vi "fgv_status-display.vi"(7 "Mode":T1=enum."Update", 8 "error in":errorcluster, 9 "detail":string, 10 "title":string, 11 "System Log":refnum<vi>) -> (0 "error out":errorcluster)   [LabVIEW 2019]
uses:
  _ctrl/system-status.ctl
panel:
  out "deleted portion":string[](array[string])
  out "concatenated string":string
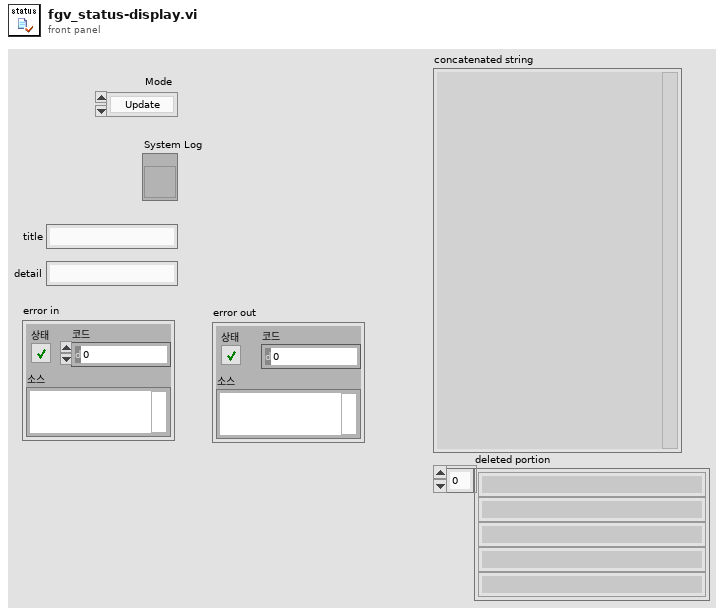
[diagram p1: front panel]
types:
  T1 = typedef "system-status.ctl" = enum16{"Initial", "Update", "Clear", "Read"}
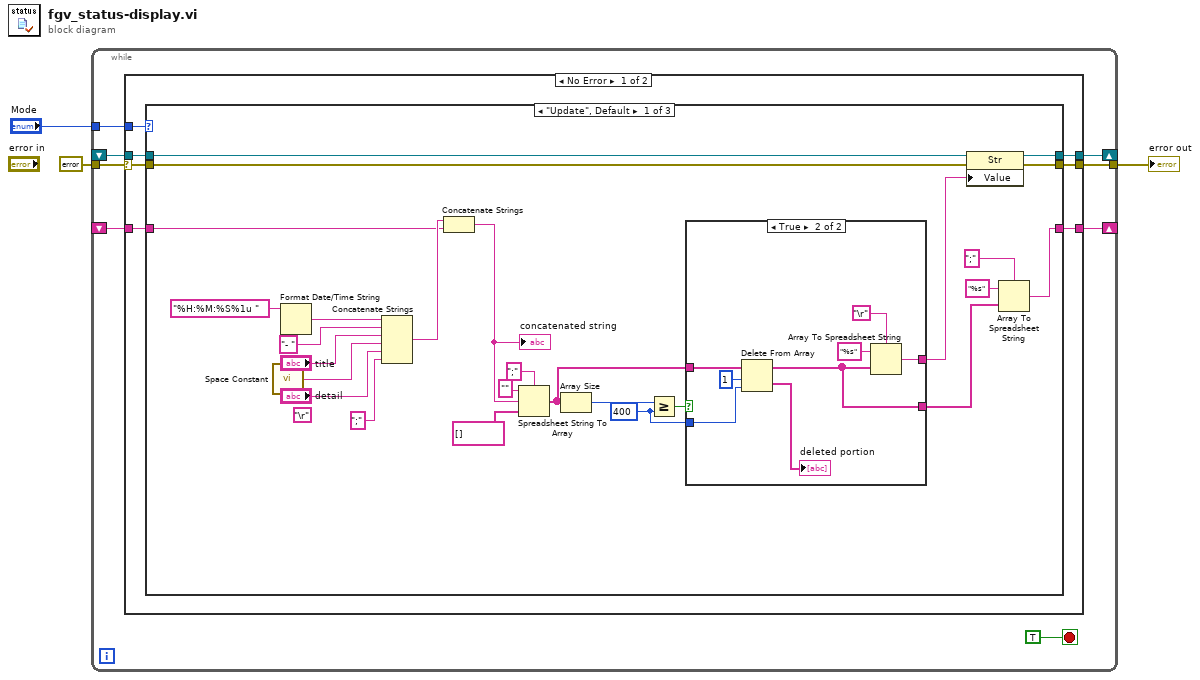
[diagram p0: block diagram]
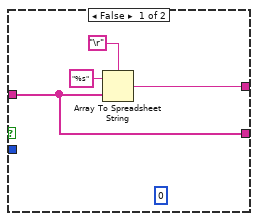
[diagram p2: hidden frame]
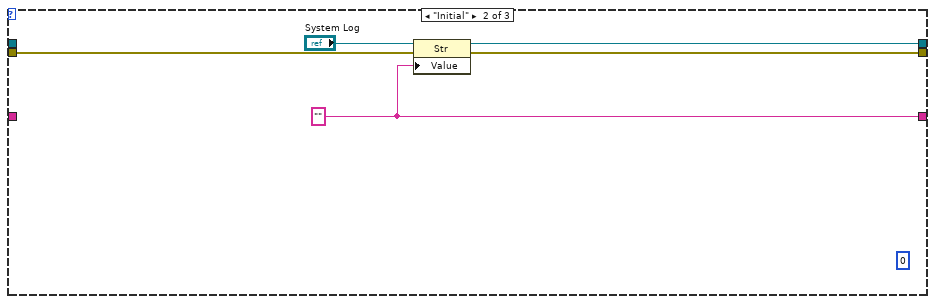
[diagram p3: hidden frame]
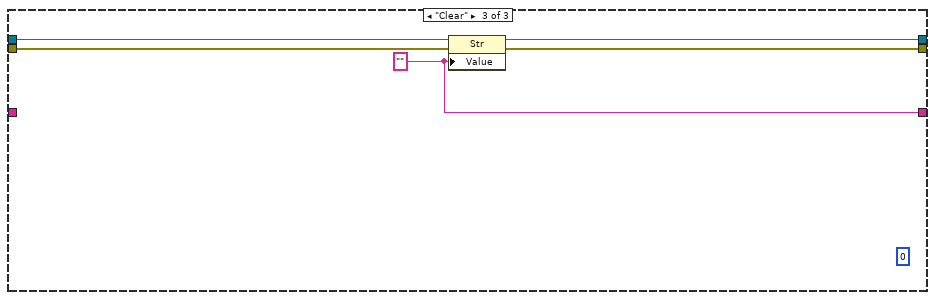
[diagram p4: hidden frame]
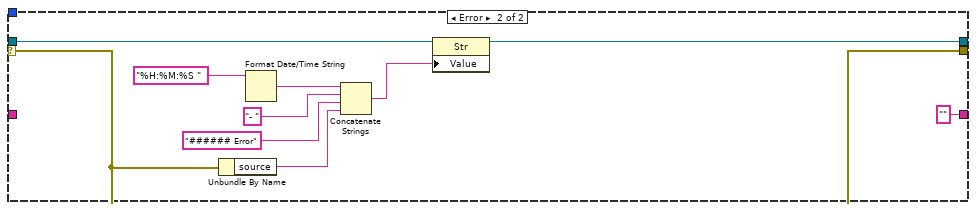
[diagram p5: hidden frame]
diagram:
  n1 = while {
    tunnel: errorcluster {"status"=FALSE, "code"=0, "source"=""} ("error in") -> [w6]
    tunnel: [w11] -> w3
    tunnel: "Mode" -> [w9]
    shift-right: [w8] -> _
    shift-left: _ -> [w7]
    shift-right: [w5] -> _
    shift-left: _ -> [w4]
    stop <- TRUE stop-if-true
    n2 = case shown="No Error" w6 {
      selector: w6 -> [w14 w68]
      tunnel: [w18 w68] -> w11
      tunnel: w9 -> [w17 _]
      tunnel: [w16 w75] -> w8
      tunnel: w7 -> [w15 w76]
      tunnel: [w13 "" ("값")] -> w5
      tunnel: w4 -> [w12 _]
      frame No Error {
        n3 = case shown="\"Update\", Default" w17 {
          tunnel: w15 -> [w25 _ w64]
          tunnel: w14 -> [w24 w59 w66]
          tunnel: [w44 w60 w65] -> w18
          tunnel: [w43 w61 w63] -> w16
          tunnel: [w19 w57 w62] -> w13
          tunnel: w12 -> [w23 _ _]
          frame "Update", Default {
            (unwired) "\r"
            w28 = 400 ("y")
            n4 = call <vilib>:"Space Constant.vi"() -> ("String"=w35:string)
            n5 = Format Date/Time String(time format string (%c)="%H:%M:%S%1u " ("시간 포맷 문자열 (%c)")) -> (date/time string=w39:string)  [unwired: 2 in]
            n6 = Concatenate Strings(w39, "- " ("포맷 문자열"), "title", w35, "detail", ";" ("string")) -> (w29:string)
            n7 = Concatenate Strings(w29, w23) -> (w30:string)
            "concatenated string" <- w30
            n8 = Spreadsheet String To Array(delimiter (Tab)=";" ("string"), format string="" ("포맷 문자열"), spreadsheet string=w30, array type (2D Dbl)=string[] []) -> (array=w32:string[])
            n9 = Array Size(array=w32) -> (size(s)=w34:i32)
            n10 = Greater Or Equal?(x=w34, y=w28) -> (x >= y?=w33:bool)
            n11 = case shown="True" w33 {
              tunnel: w32 -> [w45 w56]
              tunnel: [w47 w54] -> w31
              tunnel: w28 -> [_ w52]
              tunnel: [w45 w49] -> w20
              frame False {
                (unwired) u32 0 ("Text.Scroll Position")
                n12 = Array To Spreadsheet String(delimiter (Tab)="\r", array=w45, 3:"%s" ("format string")) -> (spreadsheet string=w47:string)
              }
              frame True {
                n13 = Delete From Array(array=w56, length=1, index=w52) -> (deleted portion=→"deleted portion":string[], array with subset deleted=w49:string[])
                n14 = Array To Spreadsheet String(delimiter (Tab)="\r", array=w49, 3:"%s" ("format string")) -> (spreadsheet string=w54:string)
              }
            }
            n15 = property class="Str"(reference=w25, error in=w24, "Value"=w31) -> (reference out=w43:refnum<vi>, error out=w44:errorcluster)
            n16 = Array To Spreadsheet String(delimiter (Tab)=";" ("string"), array=w20, 3:"%s" ("format string")) -> (spreadsheet string=w19:string)
          }
          frame "Initial" {
            (unwired) u32 0 ("Text.Scroll Position")
            w57 = "" ("값")
            n17 = property class="Str"(reference="System Log", error in=w59, "Value"=w57) -> (reference out=w61:refnum<vi>, error out=w60:errorcluster)
          }
          frame "Clear" {
            (unwired) u32 0 ("Text.Scroll Position")
            w62 = "" ("값")
            n18 = property class="Str"(reference=w64, error in=w66, "Value"=w62) -> (reference out=w63:refnum<vi>, error out=w65:errorcluster)
          }
        }
      }
      frame Error {
        n19 = Unbundle By Name(w68) -> ("source"=w70:string)
        n20 = Format Date/Time String(time format string (%c)="%H:%M:%S " ("시간 포맷 문자열 (%c)")) -> (date/time string=w73:string)  [unwired: 2 in]
        n21 = Concatenate Strings(w73, "- " ("포맷 문자열"), "###### Error" ("문자열"), w70) -> (w71:string)
        n22 = property class="Str"(reference=w76, "Value"=w71) -> (reference out=w75:refnum<vi>)  [unwired: 1 in, 1 out]
      }
    }
  }
  "error out" <- w3
